vi "Log_Pictures.vi"   [LabVIEW 2022 SP3]
uses:
  Anemometry Sub Vis/Controls/Post_Process.ctl
  Anemometry Sub Vis/Globals/Preference_global.vi
  Anemometry Sub Vis/Globals/Extra_Commands_Global.vi
  Anemometry Sub Vis/Globals/Meas_global.vi
  Camera Server/Globals/CamServer global.vi
  Anemometry Sub Vis/Globals/Trav_pos_global.vi
types:
  T1 = typedef "Post_Process.ctl" = enum16{"Take New Data", "Post Process Raw Data File"}
  T2 = typedef "Camera enum.ctl" = string
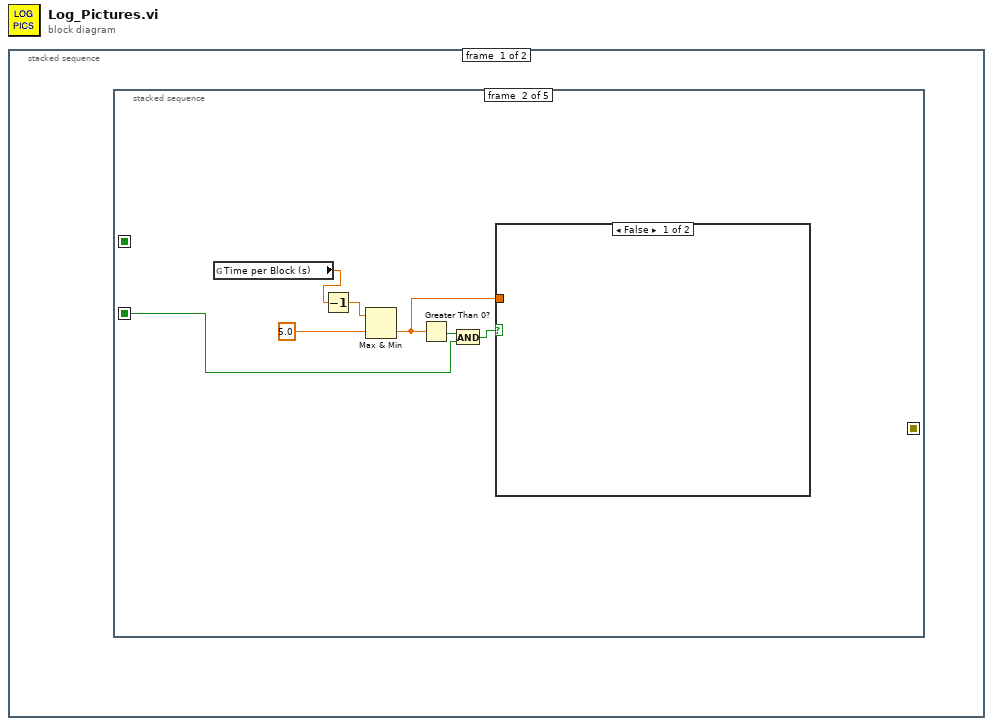
[diagram p0: block diagram]
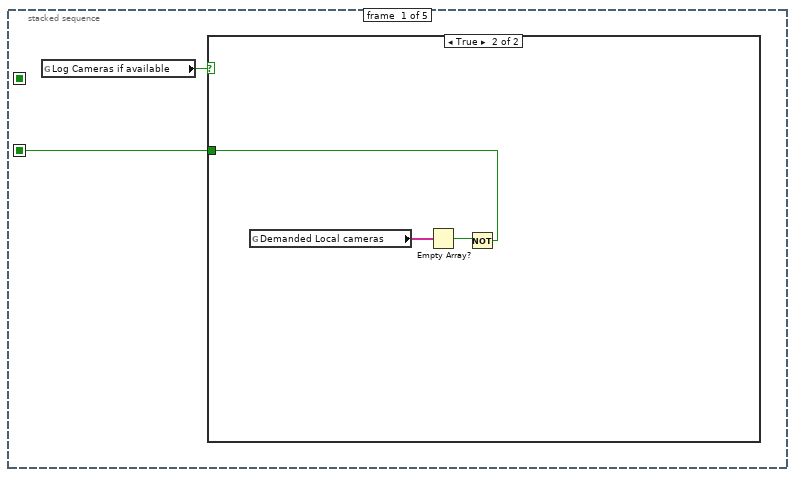
[diagram p2: hidden frame]
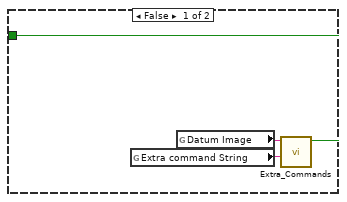
[diagram p3: hidden frame]
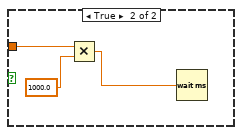
[diagram p4: hidden frame]
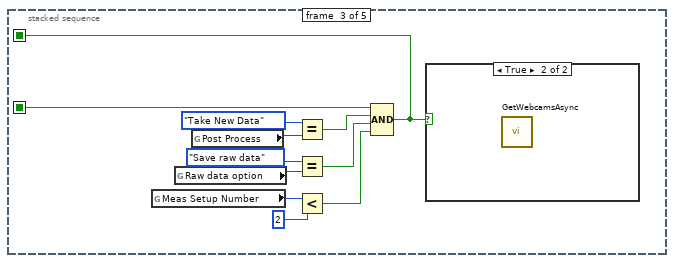
[diagram p5: hidden frame]
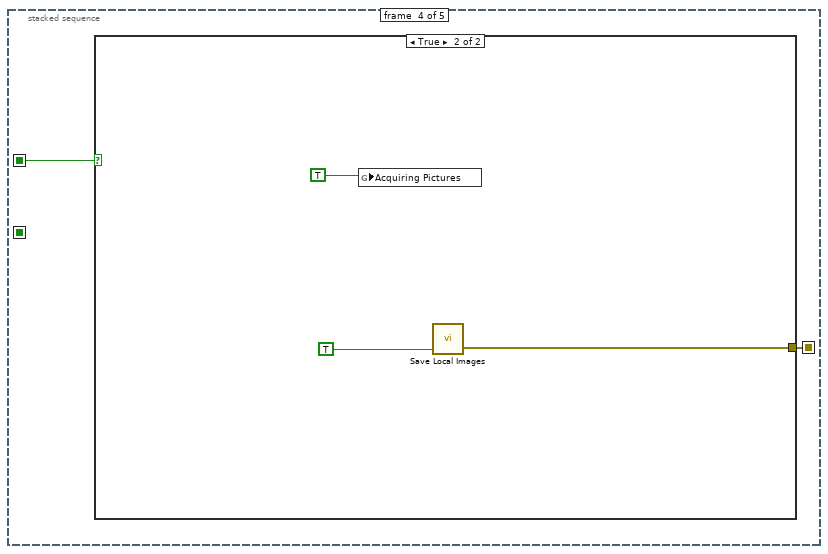
[diagram p7: hidden frame]
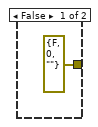
[diagram p8: hidden frame]
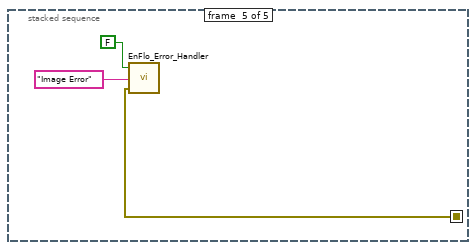
[diagram p9: hidden frame]
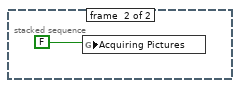
[diagram p10: hidden frame]
diagram:
  n1 = stacked-sequence {
    frame #0 {
      n2 = stacked-sequence {
        seq-local: [_ _ w19 _ _] -> [_ _ _ w31 _]
        seq-local: [w1 _ _ _ _] -> [_ w9 w20 _ _]
        seq-local: [_ _ _ w30 _] -> [_ _ _ _ w36]
        frame #0 {
          n3 = global read "Preference_global.vi" "Log Cameras if available"() -> (w2:bool)
          n4 = case shown="True" w2 {
            tunnel: [w3 w6] -> w1
            frame False {
              n5 = global read "Meas_global.vi" "Extra command String"() -> (w5:string)
              n6 = global read "Extra_Commands_Global.vi" "Datum Image"() -> (w4:string)
              n7 = call "Extra_Commands.vi"("String to Search"=w5, "Command"=w4) -> ("Command Found"=w3:bool)  [unwired: 2 in, 3 out]
            }
            frame True {
              n8 = global read "CamServer global.vi" "Demanded Local cameras"() -> (w8:T2[])
              n9 = Empty Array?(array=w8) -> (empty?=w7:bool)
              n10 = Not(x=w7) -> (.not. x?=w6:bool)
            }
          }
        }
        frame #1 {
          n11 = global read "Meas_global.vi" "Time per Block (s)"() -> (w14:dbl)
          n12 = Decrement(x=w14) -> (x-1=w13:dbl)
          n13 = Max & Min(x=w13, y=5.0) -> (min(x,y)=w12:dbl)  [unwired: 1 out]
          n14 = Greater Than 0?(x=w12) -> (x > 0?=w10:bool)
          n15 = And(x=w10, y=w9) -> (x .and. y?=w11:bool)
          n16 = case shown="False" w11 {
            tunnel: w12 -> [_ w18]
            frame False {
            }
            frame True {
              n17 = Multiply(x=w18, y=1000.0) -> (x*y=w16:dbl)
              n18 = Wait (ms)(milliseconds to wait=w16) -> ()  [unwired: 1 out]
            }
          }
        }
        frame #2 {
          n19 = global read "Trav_pos_global.vi" "Meas Setup Number"() -> (w23:i32)
          n20 = global read "Meas_global.vi" "Raw data option"() -> (w26:enum16{"Save raw data", "Raw data not saved"})
          n21 = global read "Meas_global.vi" "Post Process"() -> (w29:T1)
          n22 = Equal?(x=Post_Process."Take New Data" ("Post Process"), y=w29) -> (x = y?=w27:bool)
          n23 = Equal?(x=enum16{"Save raw data", "Raw data not saved"}."Save raw data" ("Raw data option"), y=w26) -> (x = y?=w24:bool)
          n24 = Less?(x=w23, y=2) -> (x < y?=w21:bool)
          n25 = Compound Arithmetic op=AND(w20, w27, w24, w21) -> (w19:bool)
          n26 = case shown="True" w19 {
            frame False {
            }
            frame True {
              n27 = call "GetWebcamsAsync.vi"() -> ()  [unwired: 12 in]
            }
          }
        }
        frame #3 {
          n28 = case shown="True" w31 {
            tunnel: [errorcluster {"status"=FALSE, "code"=0, "source"=""} ("Error out") w33] -> w30
            frame False {
            }
            frame True {
              n29 = global write "Meas_global.vi" "Acquiring Pictures"(TRUE) -> ()
              n30 = call "Save Local Images.vi"("Save Images"=TRUE) -> ("error out"=w33:errorcluster)  [unwired: 2 in, 1 out]
            }
          }
        }
        frame #4 {
          n31 = call "EnFlo_Error_Handler.vi"("error in (no error)"=w36, "Error Type"="Image Error", "Dialog Box (F)"=FALSE ("Dialog Box (T)")) -> ()  [unwired: 1 in, 2 out]
        }
      }
    }
    frame #1 {
      n32 = global write "Meas_global.vi" "Acquiring Pictures"(FALSE) -> ()
    }
  }
